vi "Get attributes.vi"(8 "error in (no error)":errorcluster, 11 "ICS in":refnum<class "ICS.lvclass">) -> (0 "error out":errorcluster, 1 "email settings":T1, 2 "control indices":i32[](array[numeric]), 3 "ICS out":refnum<class "ICS.lvclass">)   [LabVIEW 2018, in "ICS.lvclass"]
uses:
  ICS.lvclass
  ICS.lvclass/ICS.ctl
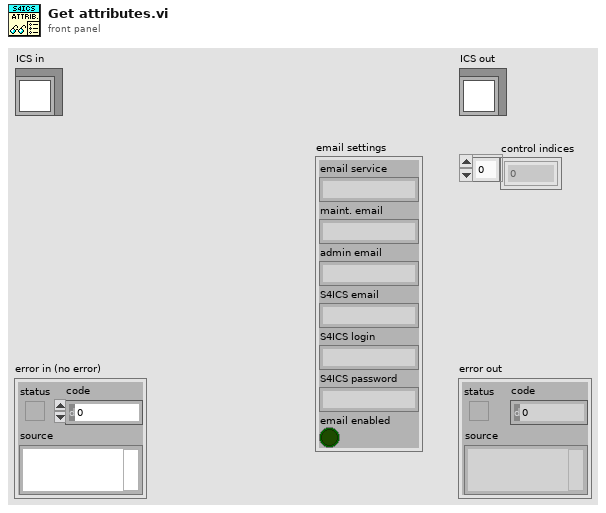
[diagram p1: front panel]
types:
  T1 = cluster{"email service":string, "maint. email":string, "admin email":string, "S4ICS email":string, "S4ICS login":string, "S4ICS password":string, "email enabled":bool}
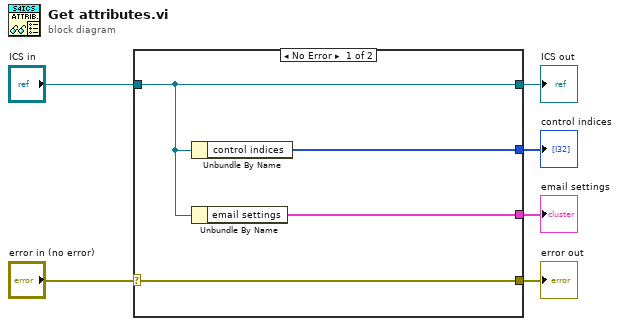
[diagram p0: block diagram]
diagram:
  n1 = case shown="No Error" "error in (no error)" {
    selector: "error in (no error)" -> [w10 w11]
    tunnel: [w10 w11] -> w5
    tunnel: [w8 w12] -> w3
    tunnel: "ICS in" -> [w8 w12]
    tunnel: [w9 _] -> w2
    tunnel: [w7 _] -> w1
    frame No Error {
      n2 = Unbundle By Name(w8) -> ("control indices"=w9:i32[])
      n3 = Unbundle By Name(w8) -> ("email settings"=w7:T1)
    }
    frame Error {
    }
  }
  "error out" <- w5
  "ICS out" <- w3
  "control indices" <- w2
  "email settings" <- w1
